vi "Main Window.vi"() -> ()   [LabVIEW 2015]
uses:
  Control Button/Exit.ctl
  Control Button/login.ctl
  Control Button/Logout.ctl
  Control Button/setting.ctl
  Control Button/report.ctl
  Control Button/Manual.ctl
  Control Button/Start.ctl
  Enqueue/Main window Seq/Test selection_1.ctl
  Enqueue/Main window Seq/Test seq_1.ctl
  Galobal variable_TI.vi
panel:
  out "Boolean 2":bool
  out "Job Id":string
  out "Error 2":bool
  out "Error":bool
  out "User Name":string
  out "error out":errorcluster
  out "x = y?":bool
  out "Company Name":string
  in  "Sign In":T1
  out "Boolean":bool
  in  "Dashbord":T6
  in  "Login Window":T8 {"User Name" items=["admin", "mmum", "a", "AJAY Kumar", "", "", "", "", "", "", "", "", "", "", "", "", "", "", "", "", "", "", "", "", "", "", "", "", "", "", "", ""]}
  in  "Exit":T9
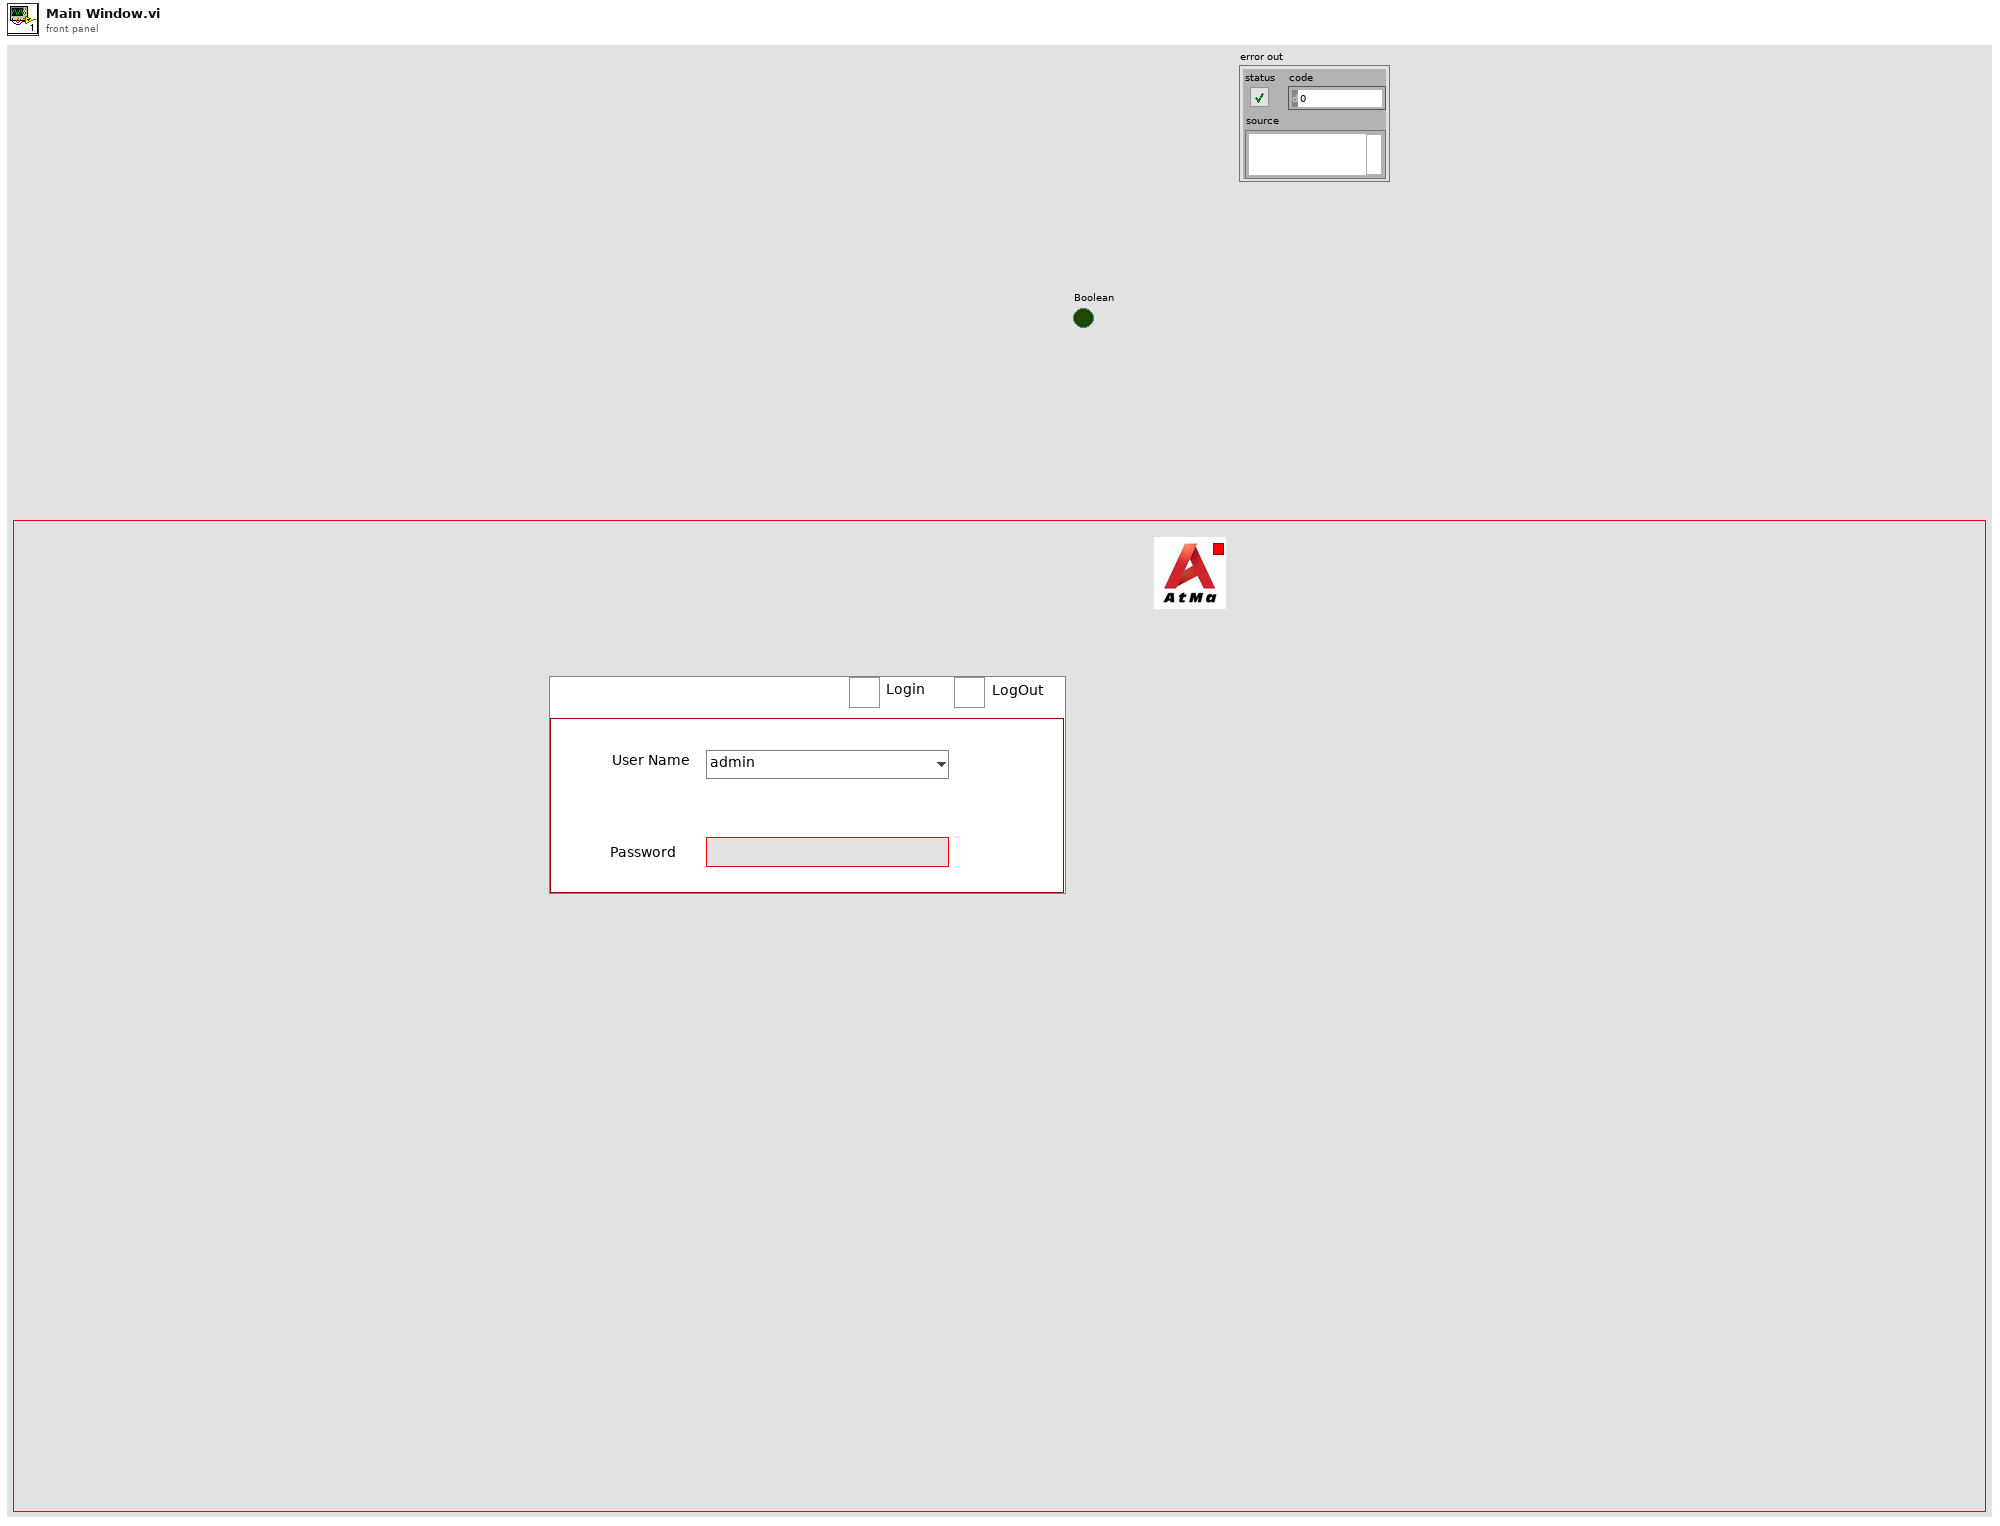
[diagram p1: front panel]
types:
  T1 = typedef "login.ctl" = bool
  T2 = typedef "setting.ctl" = bool
  T3 = typedef "report.ctl" = bool
  T4 = typedef "Manual.ctl" = bool
  T5 = typedef "Start.ctl" = bool
  T6 = cluster{"Setting":T2, "Report":T3, "Manaul":T4, "Start":T5}
  T7 = typedef "Logout.ctl" = bool
  T8 = cluster{"User Name":u16, "Password":string, "Sign In":T1, "Log Out":T7}
  T9 = typedef "Exit.ctl" = bool
  T10 = typedef "Test selection_1.ctl" = enum16{"Init", "Enqueue ", "Enqueue N", "Enqueue in stack", "Enqueue in stack N", "Dequeue", "Dequeue N", "Flush", "Release Queue"}
  T11 = typedef "Test seq_1.ctl" = enum16{"Poll Event", "Login", "Logout", "Confi", "Manual", "Report", "Testing", "Exit"}
  T12 = cluster{"XInput":dbl[], "Y New Value":dbl[], "Avg point":i16}[]
  T13 = cluster{"Slop":dbl[], "Intercept":dbl[], "Average ":i16[]}
  T14 = cluster{"UserName":string[], "Password":string[], "Usertype":string[], "Analog Min":string[], "Analog Max":string[], "DigitalInput Port":string[], "Digital Output Port":string[], "ANalog Port":string[], "IOList":cluster{"DI List_280":string[], "D0List _280":string[], "AI List_280":string[]}}
  T15 = cluster{"DI List_280":string[], "D0List _280":string[], "AI List_280":string[]}
  T16 = cluster{"DigitalInput Port[0]":string, "DigitalInput Port[1]":string, "DigitalInput Port[2]":string, "DigitalInput Port[3]":string, "DigitalInput Port[4]":string, "DigitalInput Port[5]":string, "DigitalInput Port[6]":string, "DigitalInput Port[7]":string, "DigitalInput Port[8]":string, "DigitalInput Port[9]":string, "DigitalInput Port[10]":string, "DigitalInput Port[11]":string, "DigitalInput Port[12]":string, "DigitalInput Port[13]":string, "DigitalInput Port[14]":string, "DigitalInput Port[15]":string}
  T17 = cluster{"Digital Output Port[0]":string, "Digital Output Port[1]":string, "Digital Output Port[2]":string, "Digital Output Port[3]":string, "Digital Output Port[4]":string, "Digital Output Port[5]":string, "Digital Output Port[6]":string, "Digital Output Port[7]":string, "Digital Output Port[8]":string, "Digital Output Port[9]":string, "Digital Output Port[10]":string, "Digital Output Port[11]":string, "Digital Output Port[12]":string, "Digital Output Port[13]":string, "Digital Output Port[14]":string, "Digital Output Port[15]":string, "Digital Output Port[16]":string, "Digital Output Port[17]":string, "Digital Output Port[18]":string, "Digital Output Port[19]":string, "Digital Output Port[20]":string, "Digital Output Port[21]":string, "Digital Output Port[22]":string, "Digital Output Port[23]":string, "Digital Output Port[24]":string, "Digital Output Port[25]":string, "Digital Output Port[26]":string, "Digital Output Port[27]":string, "Digital Output Port[28]":string, "Digital Output Port[29]":string}
  T18 = cluster{"ANalog Port[0]":string, "ANalog Port[1]":string, "ANalog Port[2]":string, "ANalog Port[3]":string, "ANalog Port[4]":string, "ANalog Port[5]":string, "ANalog Port[6]":string, "ANalog Port[7]":string, "ANalog Port[8]":string, "ANalog Port[9]":string, "ANalog Port[10]":string, "ANalog Port[11]":string, "ANalog Port[12]":string, "ANalog Port[13]":string, "ANalog Port[14]":string, "ANalog Port[15]":string, "ANalog Port[16]":string, "ANalog Port[17]":string, "ANalog Port[18]":string, "ANalog Port[19]":string, "ANalog Port[20]":string, "ANalog Port[21]":string, "ANalog Port[22]":string, "ANalog Port[23]":string, "ANalog Port[24]":string, "ANalog Port[25]":string, "ANalog Port[26]":string, "ANalog Port[27]":string, "ANalog Port[28]":string, "ANalog Port[29]":string, "ANalog Port[30]":string, "ANalog Port[31]":string}
  T19 = enum32{"Invalid", "Standard", "Closed", "Hidden", "Minimized", "Maximized"}
  T20 = enum8{"Enabled", "Disabled", "Disabled and Grayed Out"}
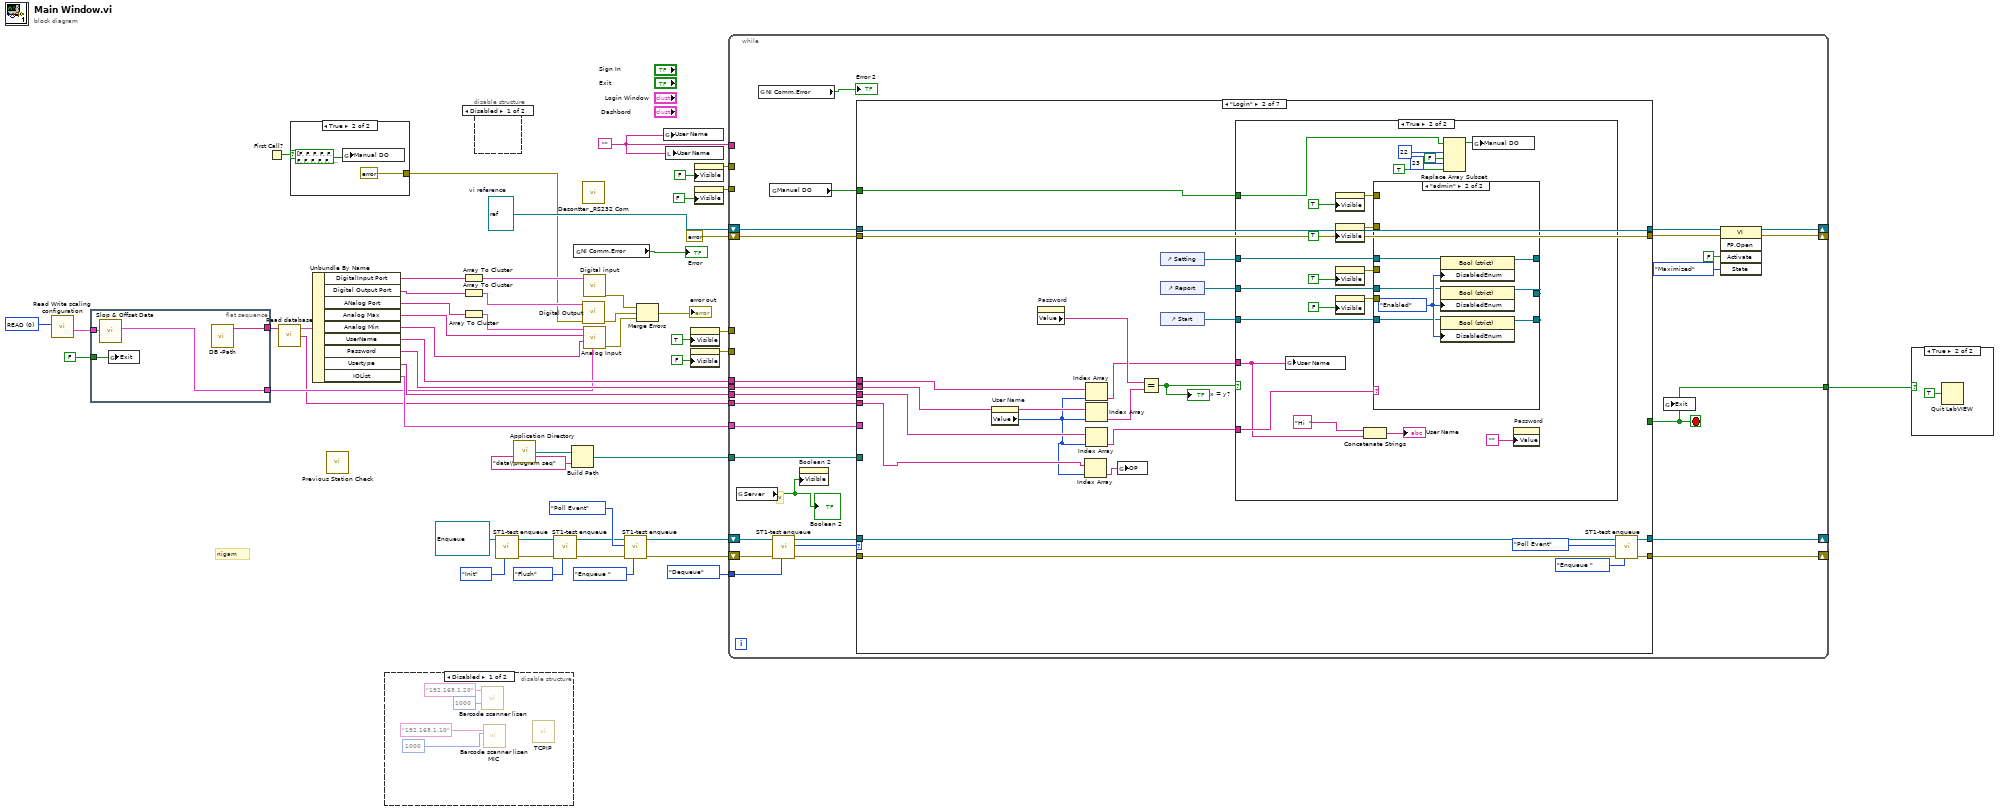
[diagram p0: block diagram]
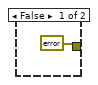
[diagram p5: hidden frame]
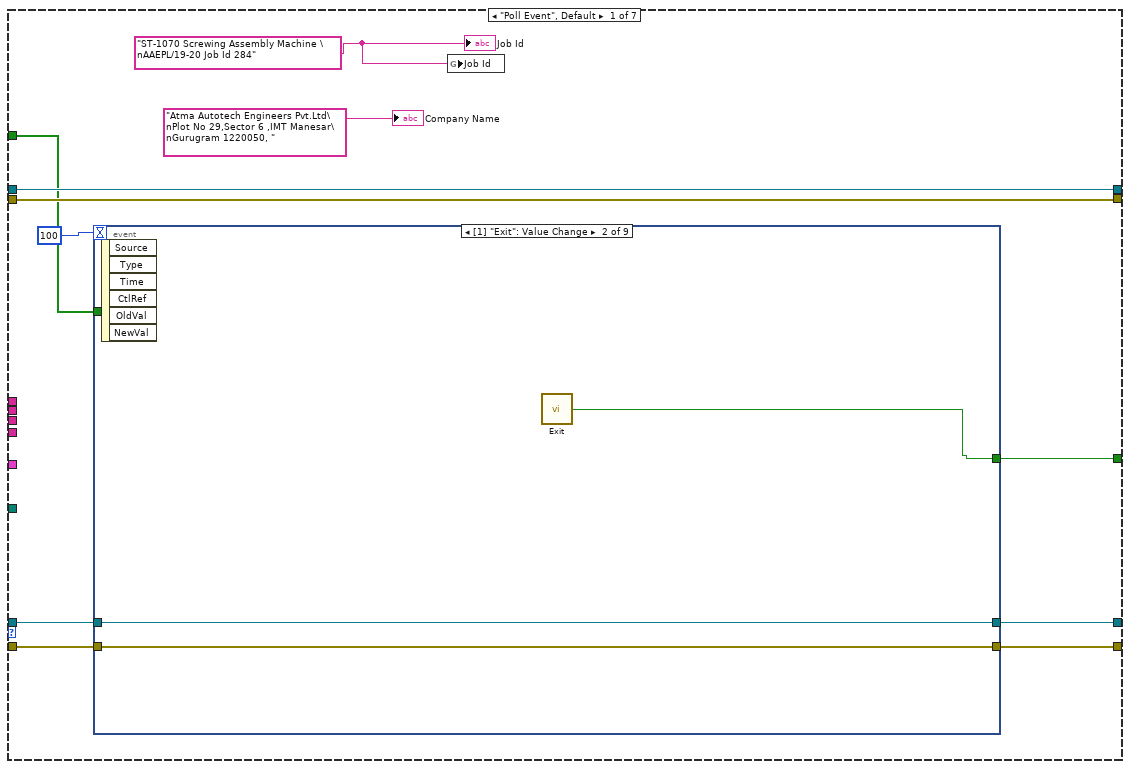
[diagram p6: hidden frame]
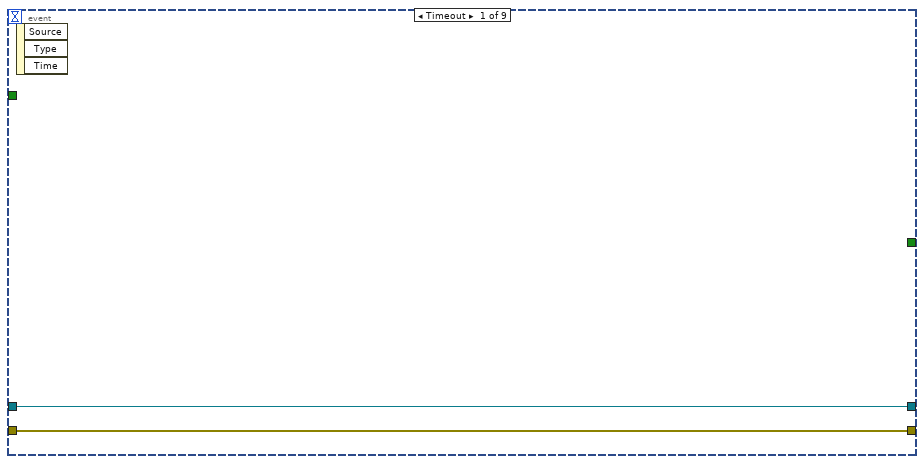
[diagram p7: hidden frame]
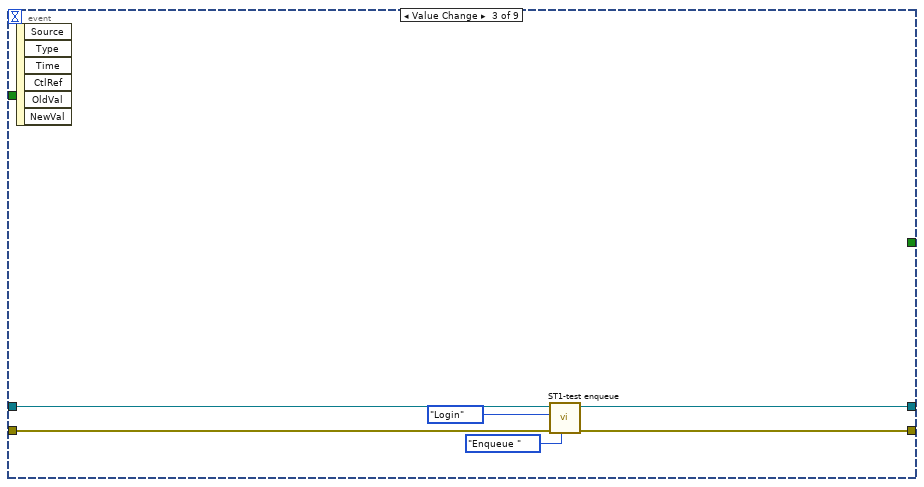
[diagram p8: hidden frame]
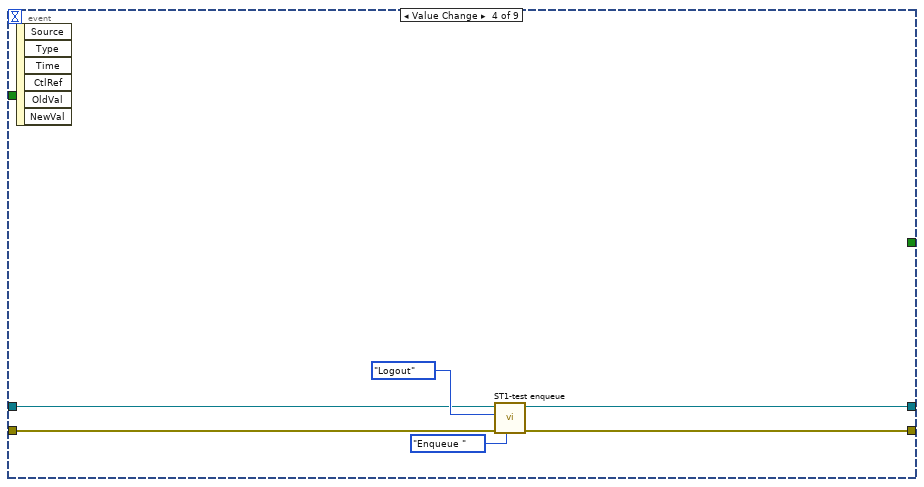
[diagram p9: hidden frame]
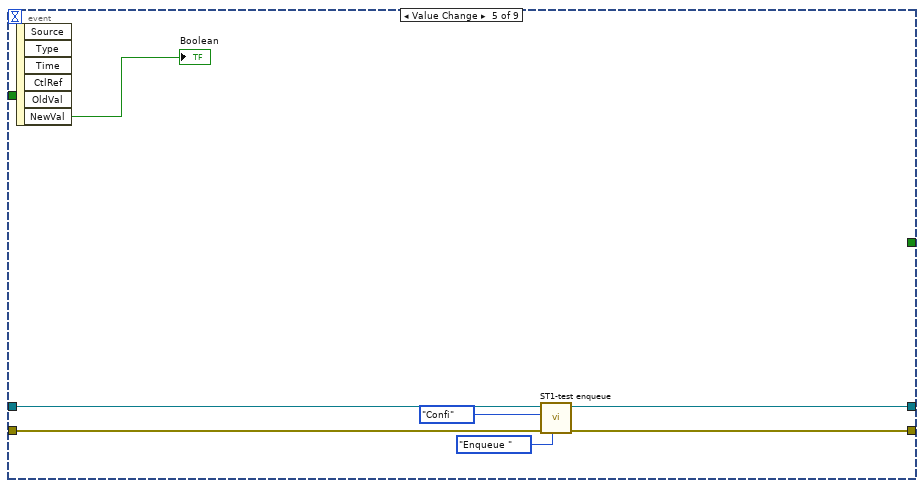
[diagram p10: hidden frame]
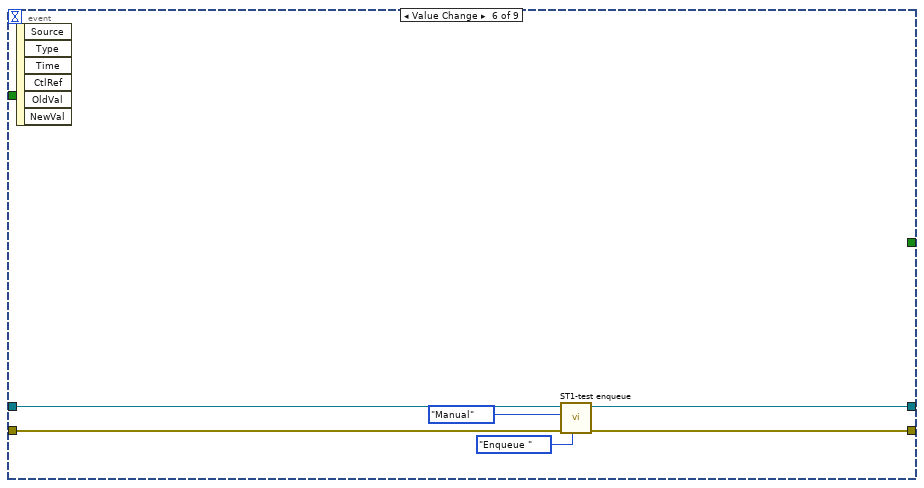
[diagram p11: hidden frame]
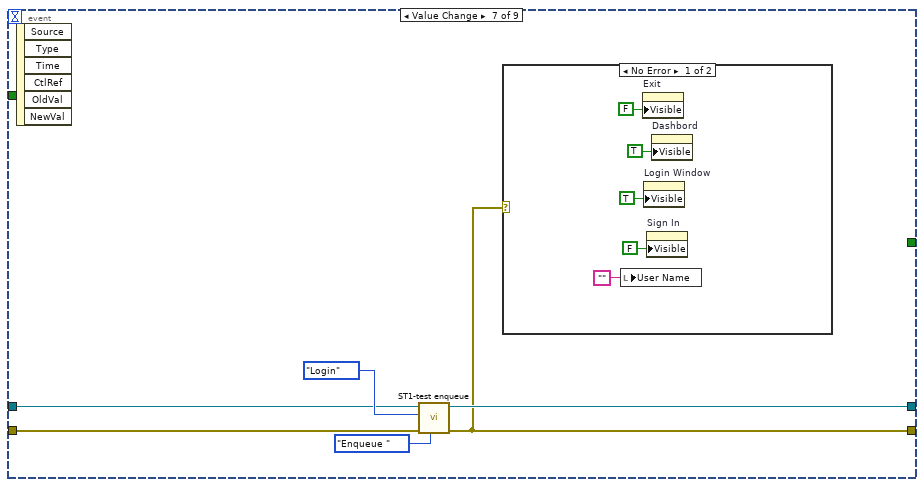
[diagram p12: hidden frame]
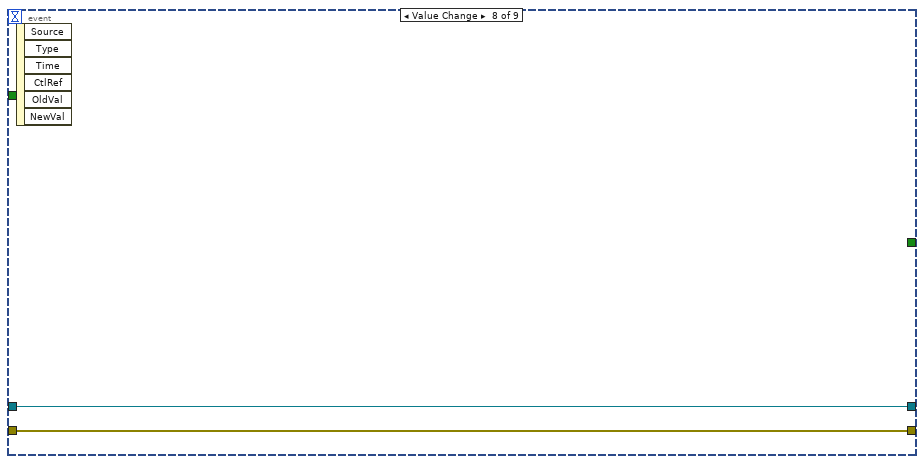
[diagram p14: hidden frame]
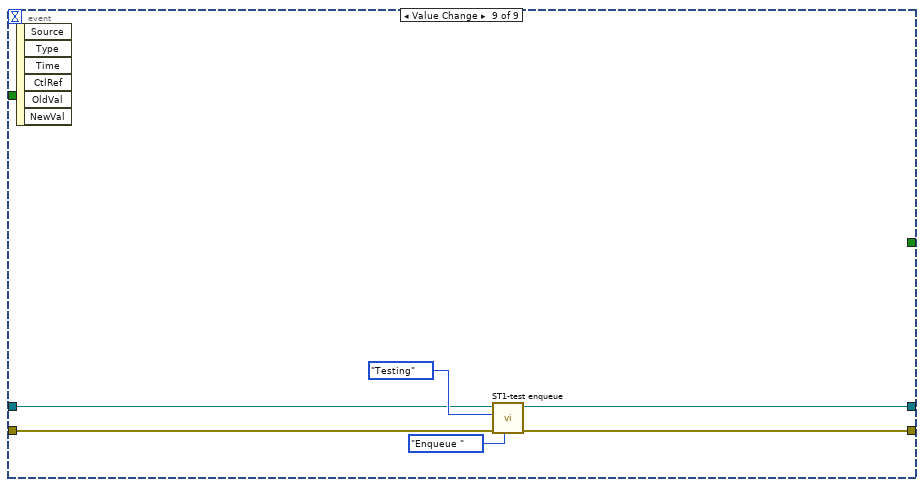
[diagram p15: hidden frame]
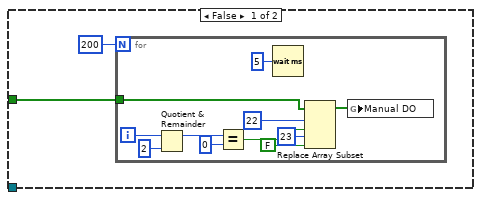
[diagram p16: hidden frame]
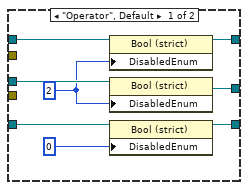
[diagram p17: hidden frame]
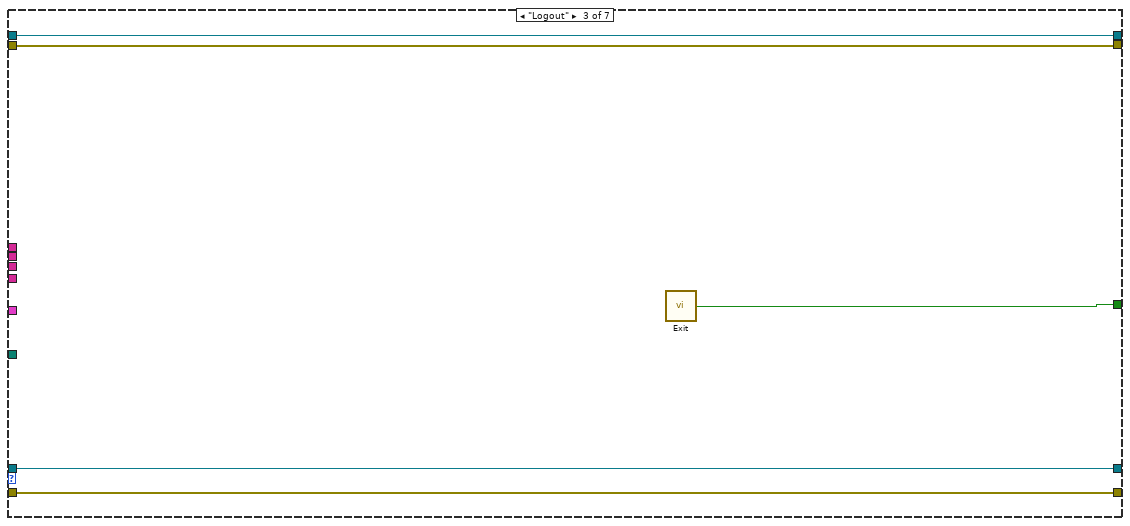
[diagram p18: hidden frame]
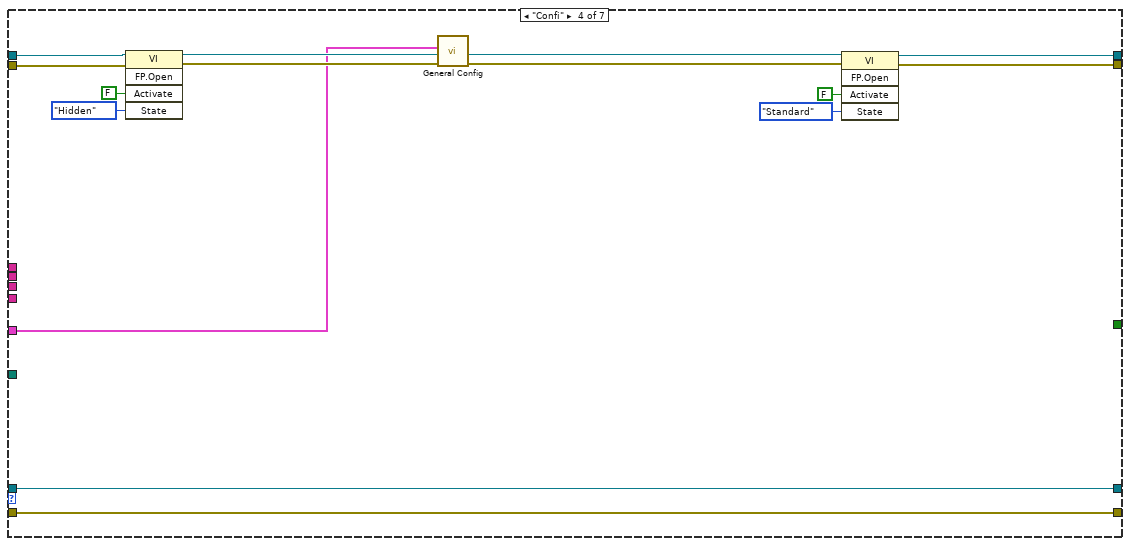
[diagram p19: hidden frame]
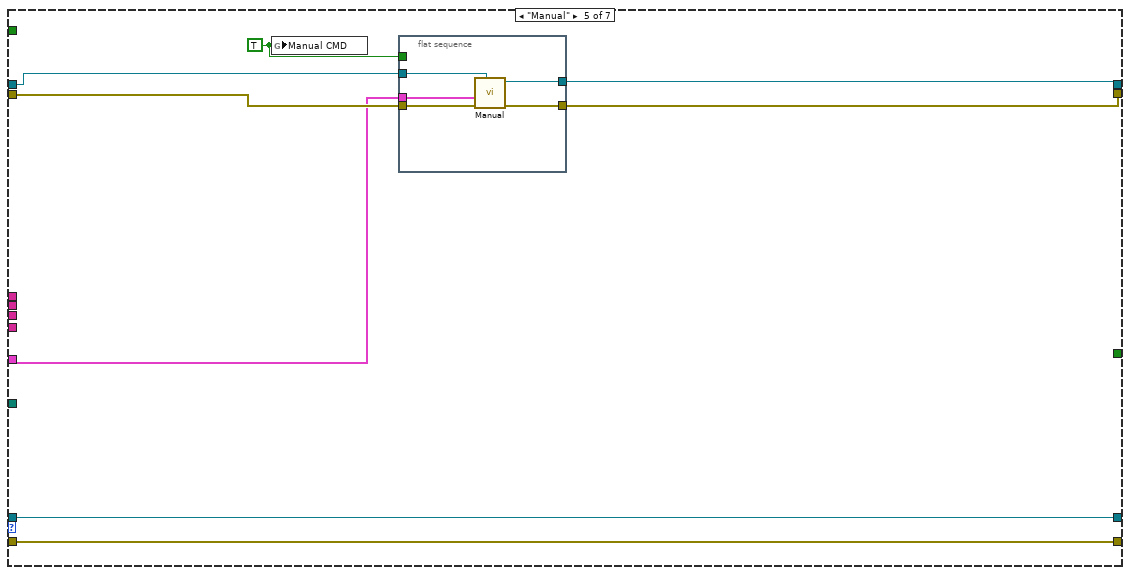
[diagram p20: hidden frame]
diagram:
  w16 = u16 0 items=["READ", "WRITE"] ("Read/Write")
  w31 = ""
  w41 = refnum<vi> refnum  # vi reference
  w42 = refnum<queue> refnum items=["Poll Event", "Login", "Logout", "Confi", "Manual", "Report", "Testing", "Exit"] ("queue in")
  # "nigam"
  n1 = call "Read Write scaling configuration.vi"("Read/Write"=w16) -> ("Output"=w15:T12)  [unwired: 4 in, 2 out]
  n2 = flat-sequence {
    tunnel: [w57] -> w30
    tunnel: w15 -> [w56]
    tunnel: [w55] -> w14
    tunnel: FALSE ("Exit") -> [w54]
    frame #0 {
      n3 = call "Slop & Offset Data.vi"("Input"=w56) -> ("Cluster"=w55:T13)  [unwired: 10 in]
      n4 = global write "Galobal variable_TI.vi" "Exit"(w54) -> ()
      n5 = call "DB -Path.vi"() -> ("String"=w57:string)  [unwired: 11 in]
    }
  }
  n6 = First Call?() -> (First Call?: T/F=w5:bool)
  n7 = call "Read database.vi"("String"=w30) -> ("Opertator id"=w1:string[], "DB Data"=w29:T14)  [unwired: 2 in, 1 out]
  n8 = case shown="True" w5 {
    tunnel: [errorcluster {"status"=FALSE, "code"=0, "source"=""} ("error constant") errorcluster {"status"=FALSE, "code"=0, "source"=""} ("error constant")] -> w4
    frame False {
    }
    frame True {
      n9 = global write "Galobal variable_TI.vi" "Manual DO"(bool[] [FALSE, FALSE, FALSE, FALSE, FALSE, FALSE, FALSE, FALSE, FALSE, FALSE, FALSE, FALSE, FALSE, FALSE, FALSE, FALSE, FALSE, FALSE, FALSE, FALSE, FALSE, FALSE, FALSE, FALSE, FALSE, FALSE, FALSE, FALSE, FALSE, FALSE] ("Manual DO")) -> ()
    }
  }
  n10 = Unbundle By Name(w29) -> ("DigitalInput Port"=w28:string[], "Digital Output Port"=w26:string[], "ANalog Port"=w24:string[], "Analog Max"=w22:string[], "Analog Min"=w21:string[], "UserName"=w20:string[], "Password"=w19:string[], "Usertype"=w18:string[], "IOList"=w17:T15)
  n11 = call "Previous Station Check.vi"() -> ()  [unwired: 12 in]
  n12 = disable-structure shown="Disabled" {
    frame Disabled {
      n13 = call "Barcode scanner lisen.vi"("port"=u16 1000, "service name"="192.168.1.20") -> ()  [unwired: 7 in, 3 out]
      n14 = call "Barcode scanner lisen MIC.vi"("port"=u16 1000, "service name"="192.168.1.10") -> ()  [unwired: 7 in, 3 out]
      n15 = call "TCPIP.vi"() -> ()  [unwired: 12 in]
    }
    frame Enabled {
    }
  }
  n16 = Array To Cluster(array=w28) -> (cluster=w27:T16)
  n17 = Array To Cluster(array=w26) -> (cluster=w25:T17)
  n18 = Array To Cluster(array=w24) -> (cluster=w23:T18)
  n19 = disable-structure shown="Disabled" {
    frame Disabled {
    }
    frame Enabled {
    }
  }
  n20 = call "ST1-test enqueue.vi"("Enum Selection"=Test_selection_1."Init", "queue in"=w42) -> ("error out"=w51:errorcluster, "queue Out"=w47:refnum<queue>)  [unwired: 6 in, 1 out]
  n21 = call <vilib>:"Application Directory.vi"() -> ("Application Directory"=w8:path)
  n22 = call "ST1-test enqueue.vi"("Enum Selection"=Test_selection_1."Flush", "Error In"=w51, "queue in"=w47) -> ("error out"=w49:errorcluster, "queue Out"=w46:refnum<queue>)  [unwired: 5 in, 1 out]
  n23 = Build Path(base path=w8, name or relative path="data\\program seq") -> (appended path=w6:path)
  n24 = global read "Galobal variable_TI.vi" "NI Comm.Error"() -> (→"Error":bool)
  n25 = call "Desontter _RS232 Com.vi"() -> ()  [unwired: 12 in]
  n26 = call "Digital Output.vi"("error in"=w4, "DAQmx OutPut Setting"=w25) -> ("error out"=w12:errorcluster)  [unwired: 8 in, 1 out]
  n27 = call "Digital input.vi"("DAQmx InPut Setting"=w27) -> ("error out"=w10:errorcluster)  [unwired: 9 in, 1 out]
  n28 = call "Analog Input.vi"("clai. Parmeter"=w14, "Min Value"=w21, "Max Value"=w22, "DAQmx Analog Input Setting"=w23) -> ("error out"=w11:errorcluster)  [unwired: 6 in, 1 out]
  n29 = call "ST1-test enqueue.vi"("Enum Selection"=Test_selection_1."Enqueue ", "Error In"=w49, "Enqueue"=Test_seq_1."Poll Event", "queue in"=w46) -> ("error out"=w44:errorcluster, "queue Out"=w45:refnum<queue>)  [unwired: 4 in, 1 out]
  n30 = Merge Errors(w10, w12, w11) -> (→"error out":errorcluster)
  n31 = global write "Galobal variable_TI.vi" "User Name"(w31) -> ()
  n32 = local write "User Name"(w31) -> ()
  n33 = property on="Login Window" class="Clust (strict)"("Visible"=TRUE) -> (error out=w36:errorcluster)  [unwired: 2 in, 1 out]
  n34 = property on="Sign In" class="Bool (strict)"("Visible"=FALSE) -> (error out=w35:errorcluster)  [unwired: 2 in, 1 out]
  n35 = property on="Exit" class="Bool (strict)"("Visible"=FALSE) -> (error out=w33:errorcluster)  [unwired: 2 in, 1 out]
  n36 = property on="Dashbord" class="Clust (strict)"("Visible"=FALSE) -> (error out=w38:errorcluster)  [unwired: 2 in, 1 out]
  n37 = while {
    shift-right: [w84] -> _
    shift-left: w45 -> [w90]
    shift-right: [w83] -> _
    shift-left: w44 -> [w89]
    tunnel: Test_selection_1."Dequeue" ("Enum Selection") -> [w88]
    shift-right: [w75] -> _
    shift-left: errorcluster {"status"=FALSE, "code"=0, "source"=""} ("error out") -> [w81]
    shift-right: [w76] -> _
    shift-left: w41 -> [w82]
    tunnel: w38 -> [_]
    tunnel: w36 -> [_]
    tunnel: w35 -> [_]
    tunnel: w33 -> [_]
    tunnel: w31 -> [_]
    tunnel: w20 -> [w74]
    tunnel: w19 -> [w73]
    tunnel: w18 -> [w72]
    tunnel: w17 -> [w71]
    tunnel: w6 -> [w70]
    tunnel: [w68] -> w3
    tunnel: w1 -> [w65]
    stop <- w68 stop-if-true
    # "v"
    n38 = global read "Galobal variable_TI.vi" "Server"() -> (w66:bool)
    "Boolean 2" <- w66
    n39 = global read "Galobal variable_TI.vi" "NI Comm.Error"() -> (→"Error 2":bool)
    n40 = global read "Galobal variable_TI.vi" "Manual DO"() -> (w69:bool[])
    n41 = call "ST1-test enqueue.vi"("Enum Selection"=w88, "Error In"=w89, "queue in"=w90) -> ("error out"=w85:errorcluster, "D-enqueue"=w87:T11, "queue Out"=w86:refnum<queue>)  [unwired: 5 in]
    n42 = property on="Boolean 2" class="Bool (strict)"("Visible"=w66) -> ()  [unwired: 2 in, 2 out]
    n43 = case shown="\"Login\"" w87 {
      tunnel: [w99 _ w224 _ _ _ _] -> w68
      tunnel: w86 -> [w100 w155 w228 w242 w250 w259 w276]
      tunnel: w85 -> [w101 w154 w227 w241 w249 w258 w275]
      tunnel: [w98 w158 w228 w242 w250 w259 w276] -> w84
      tunnel: [w97 w157 w227 w241 w249 w258 w275] -> w83
      tunnel: [w96 w167 w226 w236 w245 w257 w262] -> w78
      tunnel: [w95 w166 w225 w235 w246 w256 w260] -> w77
      tunnel: w82 -> [w96 w167 w226 w234 w247 w257 w268]
      tunnel: w81 -> [w95 w166 w225 w233 w248 w256 w271]
      tunnel: w74 -> [_ w164 _ _ _ _ _]
      tunnel: w73 -> [_ w163 _ _ _ _ _]
      tunnel: w72 -> [_ w162 _ _ _ _ _]
      tunnel: w71 -> [_ _ _ w229 w244 _ w274]
      tunnel: w70 -> [_ _ _ _ _ _ w266]
      tunnel: w69 -> [w92 w156 _ _ _ _ _]
      tunnel: w65 -> [_ w153 _ _ _ _ _]
      frame "Poll Event", Default {
        w91 = "ST-1070 Screwing Assembly Machine \nAAEPL/19-20 Job Id 284" ("string")
        n44 = event shown="[1] \"Exit\": Value Change" {
          selector: _ -> [_ _ _ _ _ _ _ _ _]
          dyn-events: _ -> [_ _ _ _ _ _ _ _ _]
          timeout: 100 -> [_ _ _ _ _ _ _ _ _]
          tunnel: [_ w104 _ _ _ _ _ _ _] -> w99
          tunnel: w101 -> [w102 w105 w110 w113 w121 w129 w135 w143 w147]
          tunnel: w100 -> [w103 w106 w111 w114 w122 w127 w134 w144 w148]
          tunnel: [w103 w106 w109 w116 w120 w126 w133 w144 w146] -> w98
          tunnel: [w102 w105 w108 w115 w119 w128 w132 w143 w145] -> w97
          tunnel: w92 -> [_ _ _ _ _ _ _ _ _]
          event Timeout {
            n45 = event-data() -> ()  [unwired: 1 in, 3 out]
          }
          event Value Change {
            n46 = event-data() -> ()  [unwired: 1 in, 6 out]
            n47 = call "Exit.vi"() -> ("Exit"=w104:bool)  [unwired: 1 in]
          }
          event Value Change {
            n48 = event-data() -> ()  [unwired: 1 in, 6 out]
            n49 = call "ST1-test enqueue.vi"("Enum Selection"=Test_selection_1."Enqueue ", "Error In"=w110, "Enqueue"=Test_seq_1."Login", "queue in"=w111) -> ("error out"=w108:errorcluster, "queue Out"=w109:refnum<queue>)  [unwired: 4 in, 1 out]
          }
          event Value Change {
            n50 = event-data() -> ()  [unwired: 1 in, 6 out]
            n51 = call "ST1-test enqueue.vi"("Enum Selection"=Test_selection_1."Enqueue ", "Error In"=w113, "Enqueue"=Test_seq_1."Logout", "queue in"=w114) -> ("error out"=w115:errorcluster, "queue Out"=w116:refnum<queue>)  [unwired: 4 in, 1 out]
          }
          event Value Change {
            n52 = event-data() -> ("NewVal"=→"Boolean":T2)  [unwired: 1 in, 5 out]
            n53 = call "ST1-test enqueue.vi"("Enum Selection"=Test_selection_1."Enqueue ", "Error In"=w121, "Enqueue"=Test_seq_1."Confi", "queue in"=w122) -> ("error out"=w119:errorcluster, "queue Out"=w120:refnum<queue>)  [unwired: 4 in, 1 out]
          }
          event Value Change {
            n54 = event-data() -> ()  [unwired: 1 in, 6 out]
            n55 = call "ST1-test enqueue.vi"("Enum Selection"=Test_selection_1."Enqueue ", "Error In"=w129, "Enqueue"=Test_seq_1."Manual", "queue in"=w127) -> ("error out"=w128:errorcluster, "queue Out"=w126:refnum<queue>)  [unwired: 4 in, 1 out]
          }
          event Value Change {
            n56 = event-data() -> ()  [unwired: 1 in, 6 out]
            n57 = call "ST1-test enqueue.vi"("Enum Selection"=Test_selection_1."Enqueue ", "Error In"=w135, "Enqueue"=Test_seq_1."Login", "queue in"=w134) -> ("error out"=w132:errorcluster, "queue Out"=w133:refnum<queue>)  [unwired: 4 in, 1 out]
            n58 = case shown="No Error" w132 {
              frame No Error {
                n59 = local write "User Name"("") -> ()
                n60 = property on="Exit" class="Bool (strict)"("Visible"=FALSE) -> ()  [unwired: 2 in, 2 out]
                n61 = property on="Login Window" class="Clust (strict)"("Visible"=TRUE) -> ()  [unwired: 2 in, 2 out]
                n62 = property on="Sign In" class="Bool (strict)"("Visible"=FALSE) -> ()  [unwired: 2 in, 2 out]
                n63 = property on="Dashbord" class="Clust (strict)"("Visible"=TRUE) -> ()  [unwired: 2 in, 2 out]
              }
              frame Error {
              }
            }
          }
          event Value Change {
            n64 = event-data() -> ()  [unwired: 1 in, 6 out]
          }
          event Value Change {
            n65 = event-data() -> ()  [unwired: 1 in, 6 out]
            n66 = call "ST1-test enqueue.vi"("Enum Selection"=Test_selection_1."Enqueue ", "Error In"=w147, "Enqueue"=Test_seq_1."Testing", "queue in"=w148) -> ("error out"=w145:errorcluster, "queue Out"=w146:refnum<queue>)  [unwired: 4 in, 1 out]
          }
        }
        n67 = global write "Galobal variable_TI.vi" "Job Id"(w91) -> ()
        "Company Name" <- "Atma Autotech Engineers Pvt.Ltd\nPlot No 29,Sector 6 ,IMT Manesar\nGurugram 1220050, " ("string")
        "Job Id" <- w91
      }
      frame "Login" {
        n68 = property on="User Name" class="Ring (strict)"() -> ("Value"=w152:u16)  [unwired: 2 in, 2 out]
        n69 = property on="Password" class="Str"() -> ("Value"=w172:string)  [unwired: 2 in, 2 out]
        n70 = Index Array(array=w153, index=w152) -> (element=w151:string)
        n71 = Index Array(array=w164, index=w152) -> (element=w165:string)
        n72 = Index Array(array=w163, index=w152) -> (element=w173:string)
        n73 = Index Array(array=w162, index=w152) -> (element=w171:string)
        n74 = global write "Galobal variable_TI.vi" "OP"(w151) -> ()
        n75 = Equal?(x=w172, y=w173) -> (x = y?=w161:bool)
        "x = y?" <- w161
        n76 = control-ref of="Setting"() -> (w170:refnum<vi>)
        n77 = control-ref of="Report"() -> (w168:refnum<vi>)
        n78 = control-ref of="Start"() -> (w169:refnum<vi>)
        n79 = case shown="True" w161 {
          tunnel: w171 -> [_ w204]
          tunnel: w170 -> [_ w208]
          tunnel: w168 -> [_ w207]
          tunnel: w169 -> [_ w206]
          tunnel: w165 -> [_ w187]
          tunnel: w156 -> [w174 w191]
          frame False {
            n80 = for {
              N: 200 -> [_]
              tunnel: w174 -> [w178]
              i -> [w186]
              n81 = Quotient & Remainder(x=w186, y=2) -> (x-y*floor(x/y)=w184:i32)  [unwired: 1 out]
              n82 = Equal?(x=w184, y=0) -> (x = y?=w181:bool)
              n83 = Wait (ms)(milliseconds to wait=u32 5) -> ()  [unwired: 1 out]
              n84 = Replace Array Subset(array=w178, new element #1=w181, index #1=22 ("index"), new element #2=FALSE ("new element/subarray"), index #2=23 ("index")) -> (w179:bool[])
              n85 = global write "Galobal variable_TI.vi" "Manual DO"(w179) -> ()
            }
          }
          frame True {
            n86 = global write "Galobal variable_TI.vi" "User Name"(w187) -> ()
            n87 = property on="Exit" class="Bool (strict)"("Visible"=TRUE) -> (error out=w195:errorcluster)  [unwired: 2 in, 1 out]
            n88 = property on="Dashbord" class="Clust (strict)"("Visible"=TRUE) -> (error out=w200:errorcluster)  [unwired: 2 in, 1 out]
            n89 = property on="Sign In" class="Bool (strict)"("Visible"=TRUE) -> (error out=w199:errorcluster)  [unwired: 2 in, 1 out]
            n90 = property on="Login Window" class="Clust (strict)"("Visible"=FALSE) -> (error out=w201:errorcluster)  [unwired: 2 in, 1 out]
            n91 = Concatenate Strings("Hi  " ("string"), w187) -> (→"User Name":string)
            n92 = case shown="\"admin\"" w204 {
              tunnel: [w216 w222] -> _
              tunnel: [w215 w221] -> _
              tunnel: [w214 w220] -> _
              tunnel: w208 -> [w213 w219]
              tunnel: w207 -> [w212 w218]
              tunnel: w206 -> [w211 w217]
              tunnel: w201 -> [_ _]
              tunnel: w200 -> [_ _]
              tunnel: w199 -> [_ _]
              tunnel: w195 -> [_ _]
              frame "Operator", Default {
                w209 = 2
                n93 = property class="Bool (strict)"(reference=w213, "DisabledEnum"=w209) -> (reference out=w216:refnum<vi>)  [unwired: 1 in, 1 out]
                n94 = property class="Bool (strict)"(reference=w212, "DisabledEnum"=w209) -> (reference out=w215:refnum<vi>)  [unwired: 1 in, 1 out]
                n95 = property class="Bool (strict)"(reference=w211, "DisabledEnum"=0) -> (reference out=w214:refnum<vi>)  [unwired: 1 in, 1 out]
              }
              frame "admin" {
                w223 = T20."Enabled" ("Disabled")
                n96 = property class="Bool (strict)"(reference=w219, "DisabledEnum"=w223) -> (reference out=w222:refnum<vi>)  [unwired: 1 in, 1 out]
                n97 = property class="Bool (strict)"(reference=w218, "DisabledEnum"=w223) -> (reference out=w221:refnum<vi>)  [unwired: 1 in, 1 out]
                n98 = property class="Bool (strict)"(reference=w217, "DisabledEnum"=w223) -> (reference out=w220:refnum<vi>)  [unwired: 1 in, 1 out]
              }
            }
            n99 = Replace Array Subset(array=w191, new element #1=FALSE ("new element/subarray"), index #1=22 ("index"), new element #2=TRUE ("new element/subarray"), index #2=23 ("index")) -> (w192:bool[])
            n100 = global write "Galobal variable_TI.vi" "Manual DO"(w192) -> ()
            n101 = property on="Password" class="Str"("Value"="") -> ()  [unwired: 2 in, 2 out]
          }
        }
        n102 = call "ST1-test enqueue.vi"("Enum Selection"=Test_selection_1."Enqueue ", "Error In"=w154, "Enqueue"=Test_seq_1."Poll Event", "queue in"=w155) -> ("error out"=w157:errorcluster, "queue Out"=w158:refnum<queue>)  [unwired: 4 in, 1 out]
      }
      frame "Logout" {
        n103 = call "Exit.vi"() -> ("Exit"=w224:bool)  [unwired: 1 in]
      }
      frame "Confi" {
        n104 = invoke class="VI" method="FP.Open"(reference=w234, error in=w233, "Activate"=FALSE ("Activate?"), "State"=T19."Hidden") -> (reference out=w230:refnum<vi>, error out=w232:errorcluster)  [unwired: 1 in, 3 out]
        n105 = call "General Config.vi"("error In"=w232, "IOList"=w229) -> ("error out"=w231:errorcluster)  [unwired: 8 in, 1 out]
        n106 = invoke class="VI" method="FP.Open"(reference=w230, error in=w231, "Activate"=FALSE ("Activate?"), "State"=T19."Standard") -> (reference out=w236:refnum<vi>, error out=w235:errorcluster)  [unwired: 1 in, 3 out]
      }
      frame "Manual" {
        w243 = TRUE ("Manual CMD")
        n107 = global write "Galobal variable_TI.vi" "Manual CMD"(w243) -> ()
        n108 = flat-sequence {
          tunnel: w248 -> [w255]
          tunnel: w247 -> [w254]
          tunnel: [w253] -> w246
          tunnel: [w252] -> w245
          tunnel: w244 -> [w251]
          tunnel: w243 -> [_]
          frame #0 {
            n109 = call "Manual.vi"("vi reference"=w254, "error in (no error)"=w255, "IOList_280"=w251) -> ("error out"=w253:errorcluster, "Out reference"=w252:refnum<vi>)  [unwired: 7 in]
          }
        }
      }
      frame "Report" {
      }
      frame "Testing" {
        n110 = Unbundle By Name(w274) -> ("DI List_280"=w267:string[])
        n111 = invoke class="VI" method="FP.Open"(reference=w268, error in=w271, "Activate"=FALSE ("Activate?"), "State"=T19."Hidden") -> (reference out=w270:refnum<vi>, error out=w269:errorcluster)  [unwired: 1 in, 3 out]
        n112 = call "Program list Selection.vi"("error in"=w269, "FeedBack Channel"=w267, "Filepath"=w266, "vi referenceIn"=w270) -> ("error out"=w261:errorcluster, "vi reference Out"=w263:refnum<vi>)  [unwired: 4 in, 2 out]
        n113 = invoke class="VI" method="FP.Open"(reference=w263, error in=w261, "Activate"=FALSE ("Activate?"), "State"=T19."Standard") -> (reference out=w262:refnum<vi>, error out=w260:errorcluster)  [unwired: 1 in, 3 out]
      }
    }
    n114 = global write "Galobal variable_TI.vi" "Exit"(w68) -> ()
    n115 = invoke class="VI" method="FP.Open"(reference=w78, error in=w77, "Activate"=FALSE ("Activate?"), "State"=T19."Maximized") -> (reference out=w76:refnum<vi>, error out=w75:errorcluster)  [unwired: 1 in, 3 out]
  }
  n116 = case shown="True" w3 {
    frame False {
    }
    frame True {
      n117 = Quit LabVIEW(quit? (T)=TRUE) -> ()
    }
  }
